vi "UHR-Fleezers Control (host) - 11.0.vi"() -> ()   [LabVIEW 2011] (continued)
        n1876 = property on="Trap Pos FB SP 2" class="DigNum (strict)"("Val(Sgnl)"=w2723) -> ()  [unwired: 2 in, 2 out]
        n1877 = local write "Offset SP2 from SP1"(FALSE ("Offset SP2 from SP1")) -> ()
      }
      event "Set Reading to\nSetpoint": Value Change {
        # "This is the actual PID input signal"
        n1878 = event-data() -> ()  [unwired: 7 out]
        n1879 = local write "Set Reading to\nSetpoint"(FALSE ("Set SP to Reading")) -> ()
        n1880 = xnode "Read/Write Control"("FPGA VI Reference In"=w2731, "error in"=w2730) -> ("FPGA VI Reference Out"=w2729:T19, "error out"=w2728:errorcluster, "Trap Pos FB Int-Norm Signal"=w2727:fxp<+/-,16,1>)
        n1881 = local read "Differential FB?"() -> (w2732:bool)
        n1882 = case shown="False" w2732 {
          tunnel: [w2737 w2744] -> w2734
          tunnel: w2727 -> [w2735 w2744]
          frame False {
            n1883 = local read "Trap Pos FB Monitor\nT1 or T2"() -> (w2740:bool)
            n1884 = local read "Trap X AI1 (DMA)"() -> (w2743:T13)
            n1885 = Unbundle By Name(w2743) -> ("Set 1"=w2742:fxp<+/-,16,1>, "Set 2"=w2741:fxp<+/-,16,1>)
            n1886 = Select(t=w2742, s=w2740, f=w2741) -> (s? t:f=w2739:fxp<+/-,16,1>)
            n1887 = Not(x="Set SP Using...") -> (.not. x?=w2736:bool)
            n1888 = Select(t=w2735, s=w2736, f=w2739) -> (s? t:f=w2737:fxp<+/-,16,1>)
          }
          frame True {
          }
        }
        n1889 = xnode "Read/Write Control"("FPGA VI Reference In"=w2729, "error in"=w2728, "Trap Pos. FB SP"=w2734) -> ()  [unwired: 2 out]
        n1890 = local write "Trap Pos FB SP"(w2734) -> ()
      }
      event "Trap Pos. FB Out Scale 2^n": Value Change {
        n1891 = event-data() -> ()  [unwired: 7 out]
        n1892 = Scale By Power Of 2(n="Trap Pos. FB Out Scale 2^n", x=ext 1.0) -> (x*2^n=w2745:ext)
        n1893 = property on="Trap Pos. FB Mult Factor" class="DigNum (strict)"("Val(Sgnl)"=w2745) -> ()  [unwired: 2 in, 2 out]
      }
      event "Trap Pos FB Int Count": Value Change {
        n1894 = event-data() -> ()  [unwired: 7 out]
        n1895 = xnode "Read/Write Control"("FPGA VI Reference In"=w2750, "error in"=w2749, "Trap Pos FB Int Count"="Trap Pos FB Int Count") -> ()  [unwired: 2 out]
      }
    }
    "error out 2" <- w1655
    n1896 = node-c288() -> ()  [unwired: 2 out]
  }
  n1897 = timed-loop "Mouse control: trap position (AOM deflection), set confocal spot from image" {
    tunnel: [w2752] -> w182
    tunnel: w1 -> [w2751]
    timing: w94 -> [_]
    timing-out: [_] -> w93
    stop <- w2752 stop-if-true
    n1898 = node-c288() -> ()  [unwired: 2 out]
    n1899 = event shown="[0] \"Pane\": Mouse Down" {
      selector: _ -> [_ _]
      dyn-events: _ -> [_ _]
      timeout: _ -> [_ _]
      tunnel: w2751 -> [w2755 _]
      event Mouse Down {
        n1900 = event-data() -> ("Time"=w2757:u32, "Coords"=w2756:T7, "Button"=w2758:u16)  [unwired: 6 out]
        n1901 = case shown="1" w2758 {
          tunnel: w2757 -> [_ _ w2864]
          tunnel: w2756 -> [_ w2795 w2862]
          tunnel: w2755 -> [_ _ w2860]
          frame 0, Default {
          }
          frame 1 {
            n1902 = property on="APD 2" class="ImageControl"() -> ("Displayed Image Position"=w2765:cluster{"Left":i32, "Top":i32})  [unwired: 2 in, 2 out]
            n1903 = property on="APD 1" class="ImageControl"() -> ("Displayed Image Position"=w2794:cluster{"Left":i32, "Top":i32})  [unwired: 2 in, 2 out]
            n1904 = property on="Detection Laser X" class="ImageControl"() -> ("Displayed Image Position"=w2791:cluster{"Left":i32, "Top":i32})  [unwired: 2 in, 2 out]
            n1905 = property on="Detection Laser Y" class="ImageControl"() -> ("Displayed Image Position"=w2790:cluster{"Left":i32, "Top":i32})  [unwired: 2 in, 2 out]
            n1906 = property on="APD 2" class="ImageControl"() -> ("Displayed Image Size"=w2764:cluster{"Width":u32, "Height":u32})  [unwired: 2 in, 2 out]
            n1907 = property on="APD 1" class="ImageControl"() -> ("Displayed Image Size"=w2792:cluster{"Width":u32, "Height":u32})  [unwired: 2 in, 2 out]
            n1908 = property on="Detection Laser X" class="ImageControl"() -> ("Displayed Image Size"=w2793:cluster{"Width":u32, "Height":u32})  [unwired: 2 in, 2 out]
            n1909 = property on="Detection Laser Y" class="ImageControl"() -> ("Displayed Image Size"=w2789:cluster{"Width":u32, "Height":u32})  [unwired: 2 in, 2 out]
            n1910 = Unbundle By Name(w2764) -> ("Width"=w2761:u32, "Height"=w2760:u32)
            n1911 = Unbundle By Name(w2765) -> ("Left"=w2763:i32, "Top"=w2762:i32)
            n1912 = Unbundle By Name(w2792) -> ("Width"=w2786:u32, "Height"=w2785:u32)
            n1913 = Unbundle By Name(w2793) -> ("Width"=w2782:u32, "Height"=w2781:u32)
            n1914 = Unbundle By Name(w2789) -> ("Width"=w2778:u32, "Height"=w2777:u32)
            n1915 = Unbundle By Name(w2794) -> ("Left"=w2788:i32, "Top"=w2787:i32)
            n1916 = Unbundle By Name(w2791) -> ("Left"=w2784:i32, "Top"=w2783:i32)
            n1917 = Unbundle By Name(w2790) -> ("Left"=w2780:i32, "Top"=w2779:i32)
            n1918 = Bundle("Left"=w2763, "Top"=w2762, "Width"=w2761, "Height"=w2760) -> (w2759:T29)  [unwired: 1 in]
            n1919 = Bundle("Left"=w2788, "Top"=w2787, "Width"=w2786, "Height"=w2785) -> (w2776:T29)  [unwired: 1 in]
            n1920 = Bundle("Left"=w2784, "Top"=w2783, "Width"=w2782, "Height"=w2781) -> (w2775:T29)  [unwired: 1 in]
            n1921 = Bundle("Left"=w2780, "Top"=w2779, "Width"=w2778, "Height"=w2777) -> (w2774:T29)  [unwired: 1 in]
            n1922 = Build Cluster Array(w2759, w2776, w2775, w2774) -> (w2773:T30)
            n1923 = for {
              tunnel: w2795 -> [w2806]
              tunnel: w2773 -> [w2807] mode=indexing
              shift-right: [w2804] -> w2771
              shift-left: TRUE -> [w2805]
              shift-right: [w2803] -> w2769
              shift-left: _ -> [w2799]
              shift-right: [w2802] -> w2768
              shift-left: _ -> [w2798]
              shift-right: [w2801] -> w2767
              shift-left: _ -> [w2797]
              shift-right: [w2800] -> w2766
              shift-left: _ -> [w2796]
              n1924 = case shown="True" w2805 {
                selector: w2805 -> [w2812 _]
                tunnel: w2807 -> [_ w2821]
                tunnel: w2806 -> [_ w2819]
                tunnel: [w2812 w2817] -> w2804
                tunnel: [w2811 w2816] -> w2803
                tunnel: [w2810 w2815] -> w2802
                tunnel: [w2809 w2814] -> w2801
                tunnel: [w2808 w2813] -> w2800
                tunnel: w2799 -> [w2811 _]
                tunnel: w2798 -> [w2810 _]
                tunnel: w2797 -> [w2809 _]
                tunnel: w2796 -> [w2808 _]
                frame False {
                }
                frame True {
                  n1925 = Unbundle(w2821) -> (w2820:T29)
                  n1926 = call "isclickinwindow.vi"("Image Param"=w2820, "Point32"=w2819) -> ("4 Y"=w2813:i32, "3 Height"=w2814:i32, "2 X"=w2815:i32, "1 Width"=w2816:i32, "In image?"=w2818:bool)  [unwired: 1 in]
                  n1927 = Not(x=w2818) -> (.not. x?=w2817:bool)
                }
              }
            }
            n1928 = Not(x=w2771) -> (.not. x?=w2770:bool)
            n1929 = case shown="True" w2770 {
              tunnel: w2768 -> [_ w2835]
              tunnel: w2766 -> [_ w2834]
              tunnel: w2769 -> [_ w2833]
              tunnel: w2767 -> [_ w2832]
              frame False {
              }
              frame True {
                w2822 = FALSE ("Get Point")
                n1930 = local read "Scan lines (y)"() -> (w2837:u64)
                n1931 = disable-structure shown="Disabled" {
                  frame Disabled {
                  }
                  frame Enabled {
                  }
                }
                n1932 = local read "Actual MCL Inc (V)"() -> (w2831:dbl)
                n1933 = local read "Scan steps (MCL)"() -> (w2836:u64)
                n1934 = Divide "Y Pix/step"(x=w2832, y=w2837) -> (x/y=w2844:dbl)
                n1935 = Divide "Y V/pix"(x=w2831, y=w2844) -> (x/y=w2843:dbl)
                n1936 = Divide "Y half step offset"(x=w2831, y=2.0) -> (x/y=w2845:dbl)
                n1937 = Divide "X pix/step"(x=w2833, y=w2836) -> (x/y=w2842:dbl)
                n1938 = Negate(x=w2845) -> (-x=w2846:dbl)
                n1939 = local read "Initial Y"() -> (w2852:dbl)
                n1940 = Multiply(x=w2834, y=w2843) -> (x*y=w2853:dbl)
                n1941 = Divide "X half step offset"(x=w2831, y=2.0) -> (x/y=w2839:dbl)
                n1942 = Divide "X V/pix"(x=w2831, y=w2842) -> (x/y=w2841:dbl)
                n1943 = Multiply(x=w2831, y=w2836) -> (x*y=w2848:dbl)
                n1944 = Compound Arithmetic op=ADD(w2846, w2853, w2852) -> (w2823:dbl)
                "Pointer Y (V)" <- w2823
                n1945 = Multiply(x=w2841, y=w2835) -> (x*y=w2850:dbl)
                n1946 = Negate(x=w2839) -> (-x=w2838:dbl)
                n1947 = local read "Initial X"() -> (w2851:dbl)
                n1948 = Negate(x=w2850) -> (-x=w2849:dbl)
                n1949 = Compound Arithmetic op=ADD(w2838, w2848, w2851, w2849) -> (w2824:dbl)
                "Pointer X (V)" <- w2824
                n1950 = case shown="True" "Set High F Confocal Spot (X-Y)" {
                  tunnel: w2824 -> [_ w2854]
                  tunnel: w2823 -> [_ w2855]
                  frame False {
                  }
                  frame True {
                    "Confocal Y 2 (V)" <- w2855
                    "Confocal X 2 (V)" <- w2854
                  }
                }
                n1951 = Or(x="Set X Only", y="Set Confocal Spot (X-Y)") -> (x .or. y?=w2827:bool)
                n1952 = Or(x="Set Confocal Spot (X-Y)", y="Set Y Only") -> (x .or. y?=w2826:bool)
                n1953 = case shown="True" w2827 {
                  tunnel: w2824 -> [_ w2856]
                  frame False {
                  }
                  frame True {
                    n1954 = property on="AO2" class="Slide (strict)"("Val(Sgnl)"=w2856) -> ()  [unwired: 2 in, 2 out]
                    "Confocal X 1 (V)" <- w2856
                  }
                }
                n1955 = case shown="True" w2826 {
                  tunnel: w2823 -> [_ w2857]
                  frame False {
                  }
                  frame True {
                    n1956 = property on="AO1" class="Slide (strict)"("Val(Sgnl)"=w2857) -> ()  [unwired: 2 in, 2 out]
                    "Confocal Y 1 (V)" <- w2857
                  }
                }
                n1957 = local write "Set High F Confocal Spot (X-Y)"(w2822) -> ()
                n1958 = local write "Set Confocal Spot (X-Y)"(w2822) -> ()
                n1959 = local write "Set X Only"(w2822) -> ()
                n1960 = local write "Set Y Only"(w2822) -> ()
              }
            }
          }
          frame 3 {
            n1961 = local read "BD 2 Frequency 1 (MHz)"() -> (w2858:dbl)
            n1962 = local read "BD 1 Frequency 1 (MHz)"() -> (w2859:dbl)
            n1963 = local write "Manipulating Trap"(TRUE ("Manipulating Trap")) -> ()
            n1964 = local write "Coords"(T7 {"Horizontal"=0, "Vertical"=0} ("Coords")) -> ()
            n1965 = while {
              tunnel: w2864 -> [w2869]
              tunnel: w2862 -> [w2868]
              tunnel: w2860 -> [w2867]
              tunnel: w2859 -> [w2866]
              tunnel: w2858 -> [w2865]
              stop <- w2870 stop-if-true
              n1966 = event shown="[0] \"Pane\": Mouse Move" {
                selector: _ -> [_ _]
                dyn-events: _ -> [_ _]
                timeout: _ -> [_ _]
                tunnel: ["Force Manip Abort" w2934] -> w2870
                tunnel: w2869 -> [w2877 _]
                tunnel: w2868 -> [w2875 _]
                tunnel: w2867 -> [w2874 _]
                tunnel: w2866 -> [w2873 _]
                tunnel: w2865 -> [w2872 _]
                event Mouse Move {
                  n1967 = event-data() -> ("Time"=w2878:u32, "Coords"=w2879:T7)  [unwired: 3 out]
                  n1968 = Less?(x=w2878, y=w2877) -> (x < y?=w2876:bool)
                  n1969 = case "Makes sure old motion events prior to mouse click aren't used" shown="False" w2876 {
                    tunnel: w2879 -> [w2921 _]
                    tunnel: w2875 -> [w2922 _]
                    tunnel: w2874 -> [w2899 _]
                    tunnel: w2873 -> [w2895 _]
                    tunnel: w2872 -> [w2894 _]
                    frame False {
                      n1970 = Subtract(x=w2921, y=w2922) -> (x-y=w2920:T7)
                      "Coords" <- w2920
                      n1971 = local read "Y RF Frequency Limits (MHz)"() -> (w2880:T16)
                      n1972 = To Double Precision Float(number=w2920) -> (double precision float=w2919:cluster{"Horizontal":dbl, "Vertical":dbl})
                      n1973 = Multiply(x=cluster{"Horizontal":dbl, "Vertical":dbl} {"Horizontal"=-1.0, "Vertical"=1.0}, y="Manipulation Scaling") -> (x*y=w2915:cluster{"Horizontal":dbl, "Vertical":dbl})
                      n1974 = local read "X RF Frequency Limits (MHz)"() -> (w2881:T16)
                      n1975 = Multiply(x=w2919, y=w2915) -> (x*y=w2917:cluster{"Horizontal":dbl, "Vertical":dbl})
                      n1976 = Unbundle By Name(w2917) -> ("Horizontal"=w2912:dbl, "Vertical"=w2916:dbl)
                      n1977 = Unbundle By Name(w2880) -> ("Maximum"=w2883:dbl, "Minimum"=w2882:dbl)
                      n1978 = Boolean To (0,1)(Boolean="Manip. X?") -> (0, 1=w2910:i16)
                      n1979 = Boolean To (0,1)(Boolean="Manip. Y?") -> (0, 1=w2907:i16)
                      n1980 = local read "BD 1 Frequency 2 (MHz)"() -> (w2897:dbl)
                      n1981 = Multiply(x=w2916, y=w2907) -> (x*y=w2909:dbl)
                      n1982 = Multiply(x=w2910, y=w2912) -> (x*y=w2913:dbl)
                      n1983 = local read "BD 2 Frequency 2 (MHz)"() -> (w2896:dbl)
                      n1984 = Unbundle By Name(w2881) -> ("Maximum"=w2885:dbl, "Minimum"=w2884:dbl)
                      n1985 = Add(x=w2894, y=w2909) -> (x+y=w2887:dbl)
                      n1986 = Add(x=w2895, y=w2913) -> (x+y=w2889:dbl)
                      n1987 = In Range and Coerce(upper limit=w2885, x=w2889, lower limit=w2884) -> (coerced(x)=w2888:dbl)  [unwired: 1 out]
                      n1988 = In Range and Coerce(upper limit=w2883, x=w2887, lower limit=w2882) -> (coerced(x)=w2886:dbl)  [unwired: 1 out]
                      n1989 = Subtract(x=w2888, y=w2897) -> (x-y=w2906:dbl)
                      n1990 = Subtract(x=w2886, y=w2896) -> (x-y=w2905:dbl)
                      n1991 = Square(x=w2906) -> (x^2=w2904:dbl)
                      n1992 = Square(x=w2905) -> (x^2=w2903:dbl)
                      n1993 = Add(x=w2904, y=w2903) -> (x+y=w2902:dbl)
                      n1994 = Square Root(x=w2902) -> (sqrt(x)=w2898:dbl)
                      n1995 = In Range and Coerce(upper limit="Limit Max (MHz)", x=w2898, lower limit="Limit Min (MHz)") -> (In Range?=w2891:bool)  [unwired: 1 out]
                      n1996 = Not(x="Limits Enable") -> (.not. x?=w2890:bool)
                      n1997 = Or(x=w2891, y=w2890) -> (x .or. y?=w2892:bool)
                      n1998 = case shown="True" w2892 {
                        tunnel: w2899 -> [_ w2932]
                        tunnel: w2898 -> [_ w2923]
                        tunnel: w2888 -> [_ w2930]
                        tunnel: w2897 -> [_ w2929]
                        tunnel: w2886 -> [_ w2928]
                        tunnel: w2896 -> [_ w2927]
                        tunnel: w2881 -> [_ w2925]
                        tunnel: w2880 -> [_ w2924]
                        frame False {
                        }
                        frame True {
                          n1999 = local read "BD 1 Frequency 3 (MHz)"() -> (w2931:dbl)
                          n2000 = local read "BD 2 Frequency 3 (MHz)"() -> (w2926:dbl)
                          n2001 = local write "Trap Delta (MHz)"(w2923) -> ()
                          n2002 = call "set RF board frequency - interlace.vi"("Board 2 Frequency Limits"=w2924, "Board 1 Frequency Limits"=w2925, "FPGA VI Reference In"=w2932, "Board 2 Frequency 3 (MHz)"=w2926, "Board 1 Frequency 3 (MHz)"=w2931, "Board 2 Frequency 2 (MHz)"=w2927, "Board 2 Frequency 1 (MHz)"=w2928, "Board 1 Frequency 2 (MHz)"=w2929, "Board 1 Frequency 1  (MHz)"=w2930) -> ()  [unwired: 1 in, 2 out]
                          n2003 = local write "BD 2 Frequency 1 (MHz)"(w2928) -> ()
                          n2004 = local write "BD 1 Frequency 1 (MHz)"(w2930) -> ()
                        }
                      }
                    }
                    frame True {
                    }
                  }
                }
                event Mouse Up {
                  n2005 = event-data() -> ("Button"=w2933:u16)  [unwired: 8 out]
                  n2006 = case shown="3" w2933 {
                    tunnel: [FALSE TRUE] -> w2934
                    frame 0, Default {
                    }
                    frame 3 {
                      n2007 = local read "Trap Delta (MHz)"() -> (w2936:dbl)
                      n2008 = property on="Initial delta (MHz)" class="DigNum (strict)"("Val(Sgnl)"=w2936) -> ()  [unwired: 2 in, 2 out]
                      n2009 = local write "Manipulating Trap"(FALSE ("Manipulating Trap")) -> ()
                    }
                  }
                }
              }
            }
          }
        }
      }
      event Mouse Move {
        n2010 = event-data() -> ()  [unwired: 6 out]
      }
    }
    n2011 = local read "Stop All"() -> (w2752:bool)
    n2012 = node-c288() -> ()  [unwired: 2 out]
  }
  n2013 = node-c288(w91) -> ()  [unwired: 1 out]
  n2014 = node-c288(w93) -> ()  [unwired: 1 out]
  n2015 = node-c288(w78) -> ()  [unwired: 1 out]
  n2016 = flat-sequence "Video" {
    tunnel: [w2947] -> w80
    tunnel: w80 -> [w2988]
    frame #0 {
      n2017 = while {
        stop <- w2940 continue-if-true
        n2018 = call "Close Video Capture.vi"() -> ("error code OUT"=w2942:i32)
        n2019 = Equal?(x=w2942, y=0) -> (x = y?=w2940:bool)
      }
      n2020 = local write "Stop All"(FALSE ("Stop All")) -> ()
    }
    frame #1 {
      n2021 = call "DMR_Init.vi"() -> ()  [unwired: 3 out]
    }
    frame #2 {
      # "Setting the destination format to Mono8 makes sure that the image can be displayed in the intensity plot."
      n2022 = call "DMR_GetDevice.vi"("search string IN"="DE019116701") -> ("device handle OUT"=w2965:i32)  [unwired: 4 in, 2 out]
      n2023 = call "DMR_OpenDevice.vi"("device handle IN"=w2965) -> ("driver handle OUT"=w2948:i32)  [unwired: 4 out]
      n2024 = call "DMR_FindList.vi"("flags IN"=u32 0 ("flags"), "list name IN"="" ("String"), "list type IN"=T31."camera descriptions", "driver handle IN"=w2948) -> ("list handle OUT"=w2951:i32)  [unwired: 2 out]
      n2025 = call "DMR_FindList.vi"("flags IN"=u32 0 ("flags"), "list name IN"="Base", "list type IN"=T31."setting", "driver handle IN"=w2948) -> ("list handle OUT"=w2949:i32)  [unwired: 2 out]
      n2026 = call "OBJ_GetHandle.vi"("object name IN"="VideoStandard", "list handle IN"=w2951) -> ("object handle OUT"=w2945:i32)  [unwired: 3 out]
      n2027 = call "OBJ_GetHandle.vi"("object name IN"="PixelFormat", "list handle IN"=w2949) -> ("object handle OUT"=w2959:i32)  [unwired: 3 out]
      n2028 = call "OBJ_SetS.vi"("value index IN"=0, "value IN"="NTSC M", "object handle IN"=w2945) -> ()  [unwired: 2 out]
      n2029 = call "OBJ_SetS.vi"("value index IN"=0, "value IN"="Mono8" ("value"), "object handle IN"=w2959) -> ()  [unwired: 2 out]
      n2030 = call "OBJ_GetHandle.vi"("object name IN"="VideoChannel", "list handle IN"=w2949) -> ("object handle OUT"=w2955:i32)  [unwired: 3 out]
      n2031 = while {
        tunnel: [w2970] -> w2947
        tunnel: w2948 -> [w2967]
        stop <- w2968 continue-if-true
        n2032 = call "DMR_ImageRequestSingle.vi"("request control IN"=0, "driver handle IN"=w2967) -> ("error code OUT"=w2969:i32, "driver handle OUT"=w2970:i32)  [unwired: 2 out]
        n2033 = Equal To 0?(x=w2969) -> (x = 0?=w2968:bool)
      }
      n2034 = call "OBJ_SetI.vi"("value index IN"=0, "value IN"=3 ("Video channel"), "object handle IN"=w2955) -> ()  [unwired: 2 out]
    }
    frame #3 {
      w2976 = T17 0 items=["Grayscale (U8)", "Grayscale (I16)", "Grayscale (SGL)", "Complex (CSG)", "RGB (U32)", "HSL (U32)", "RGB (U64)"] ("Image Type")
      w2984 = T17 0 items=["Grayscale (U8)", "Grayscale (I16)", "Grayscale (SGL)", "Complex (CSG)", "RGB (U32)", "HSL (U32)", "RGB (U64)"] ("Image Type")
      n2035 = for "Create Greyscale map" {
        N: 256 -> [_]
        tunnel: [w2990] -> w2973 mode=indexing
        workers-P: _ -> [_]
        i -> [w2993]
        n2036 = To Unsigned Byte Integer(number=w2993) -> (unsigned 8bit integer=w2989:u8)
        n2037 = Join Numbers(hi=w2989, lo=w2989) -> ((hi.lo)=w2992:u16)
        n2038 = Join Numbers(hi=w2989, lo=w2989) -> ((hi.lo)=w2991:u16)
        n2039 = Join Numbers(hi=w2992, lo=w2991) -> ((hi.lo)=w2990:u32)
      }
      n2040 = call "IMAQ Create"("Image Name"="Scaled video", "Image Type"=w2976) -> ("New Image"=w2975:T2)  [unwired: 2 in, 2 out]
      n2041 = call "IMAQ Create"("Image Name"="Main video", "Image Type"=w2984) -> ("New Image"=w2985:T2)  [unwired: 2 in, 2 out]
      n2042 = node-c288(0 ("Processor")) -> (w2983:T21)  [unwired: 3 out]
      n2043 = Initialize Array(u32 0 ("Window Number (0...15)"), 480 ("dimension size"), 640 ("dimension size")) -> (w2978:u32[][])
      n2044 = timed-loop {
        tunnel: w2988 -> [w3010]
        tunnel: [w3009] -> w2987
        tunnel: w2985 -> [w3008]
        timing: w2983 -> [_]
        timing-out: [_] -> w2982
        tunnel: w2978 -> [w2997]
        tunnel: w2975 -> [w2995]
        tunnel: w2973 -> [w2994]
        stop <- w2996 stop-if-true
        # "This block performs the \nactual image capture."
        n2045 = node-c288() -> ()  [unwired: 2 out]
        n2046 = local read "Stop All"() -> (w2996:bool)
        n2047 = Reciprocal(x="Video Capture Rate (Hz)") -> (1/x=w3000:dbl)
        n2048 = Multiply(x=w3000, y=1000.0) -> (x*y=w2998:dbl)
        n2049 = call "DMR_ImageRequestWaitFor.vi"("queue number IN"=0, "timeout(ms) IN"=500, "driver handle IN"=w3010) -> ("error code OUT"=w3014:i32, "request number OUT"=w3011:i32, "driver handle OUT"=w3012:i32)
        n2050 = feedback #1(T32 refnum ("Avi Refnum")) -> (w3002:T32)
        n2051 = case shown="True" "New Video File" {
          tunnel: [T32 refnum ("Avi Refnum") w3031] -> w3004
          tunnel: [FALSE TRUE] -> w3005
          tunnel: w3002 -> [_ w3027]
          frame False {
          }
          frame True {
            n2052 = call "Create new save file.vi"("Ext"=".avi" ("string"), "Index In"="Video Index") -> ("Path Out"=w3023:path, "Index Out"=w3024:dbl)  [unwired: 1 in]
            "Path Out" <- w3023
            n2053 = Not Equal?(x=w3027, y=T32 refnum ("Avi Refnum")) -> (x != y?=w3028:bool)
            n2054 = Increment(x=w3024) -> (x+1=w3033:dbl)
            n2055 = case shown="True" w3028 {
              tunnel: w3027 -> [_ w3034]
              frame False {
              }
              frame True {
                n2056 = call "IMAQ AVI Close"("Avi Refnum"=w3034) -> ()  [unwired: 1 in, 10 out]
              }
            }
            n2057 = local write "Video Index"(w3033) -> ()
            n2058 = call "IMAQ AVI Create"("Frames Per Second"=u32 30, "AVI Path"=w3023) -> ("Avi Refnum"=w3031:T32)  [unwired: 5 in, 4 out]
          }
        }
        n2059 = Equal To 0?(x=w3014) -> (x = 0?=w3013:bool)
        n2060 = Select(t=w3004, s=w3005, f=w3002) -> (s? t:f=w3003:T32)
        n2061 = feedback-in #1(w3003) -> ()
        n2062 = case shown="True" w3013 {
          tunnel: w3012 -> [w3035 w3060]
          tunnel: w3011 -> [_ w3059]
          tunnel: [w3035 w3056] -> w3009
          tunnel: w3008 -> [_ w3040]
          tunnel: w2997 -> [_ w3044]
          tunnel: w3003 -> [_ w3042]
          tunnel: w2995 -> [_ w3037]
          tunnel: w2994 -> [_ w3036]
          frame False {
          }
          frame True {
            w3050 = u32 0 ("X-offset IN")
            n2063 = call "DMR_GetImageRequestBufferData.vi"("driver handle IN"=w3060, "request number IN"=w3059) -> ("width OUT"=w3049:i32, "height OUT"=w3048:i32, "driver handle OUT"=w3055:i32, "request number OUT"=w3054:i32, "bytes per pixel OUT"=w3051:i32)  [unwired: 13 out]
            n2064 = call "DMR_GetImageRequestBufferImageData.vi"("driver handle IN"=w3055, "request number IN"=w3054, "bytes per pixel IN"=w3051, "X-offset IN"=w3050, "Y-offset IN"=w3050, "height IN"=w3048, "width IN"=w3049) -> ("driver handle OUT"=w3053:u32, "request number OUT"=w3052:u32, "image OUT"=w3045:u32[][])  [unwired: 10 out]
            n2065 = call "DMR_ImageRequestUnlock.vi"("request number IN"=w3052, "driver handle IN"=w3053) -> ("driver handle OUT"=w3058:i32)  [unwired: 1 in, 2 out]
            n2066 = case shown="True" "Averaging" {
              tunnel: w3045 -> [w3096 w3101]
              tunnel: [w3096 w3100] -> w3041
              tunnel: w3044 -> [_ w3098]
              frame False {
              }
              frame True {
                (unwired) 1
                w3106 = 1
                n2067 = feedback #2(w3098) -> (w3097:u32[][])
                n2068 = Add(x=w3101, y=w3097) -> (x+y=w3102:u32[][])
                n2069 = Select(t=w3098, s="Reset Averaging", f=w3102) -> (s? t:f=w3104:u32[][])
                n2070 = feedback-in #2(w3104) -> ()
                n2071 = feedback #3(w3106) -> (w3099:i32)
                n2072 = Divide(x=w3102, y=w3099) -> (x/y=w3103:dbl[][])
                n2073 = Increment(x=w3099) -> (x+1=w3107:i32)
                n2074 = To Unsigned Long Integer(number=w3103) -> (unsigned 32bit integer=w3100:u32[][])
                n2075 = Select(t=w3106, s="Reset Averaging", f=w3107) -> (s? t:f=w3105:i32)
                n2076 = feedback-in #3(w3105) -> ()
              }
            }
            n2077 = call "DMR_ImageRequestSingle.vi"("request control IN"=0, "driver handle IN"=w3058) -> ("driver handle OUT"=w3056:i32)  [unwired: 3 out]
            n2078 = disable-structure shown="Disabled" {
              disable-tunnel: w3041 -> [w3073 _]
              disable-tunnel: w3037 -> [w3072 _]
              frame Disabled {
                n2079 = To Double Precision Float(number=w3073) -> (double precision float=w3071:dbl[][])
                n2080 = In Range and Coerce(upper limit="Intensity Upper", x=w3071, lower limit="Intensity Lower") -> (coerced(x)=w3070:dbl[][])  [unwired: 1 out]
                n2081 = Subtract(x="Intensity Upper", y="Intensity Lower") -> (x-y=w3067:dbl)
                n2082 = Subtract(x=w3070, y="Intensity Lower") -> (x-y=w3068:dbl[][])
                n2083 = Divide(x=w3068, y=w3067) -> (x/y=w3069:dbl[][])
                n2084 = Multiply(x=255.0, y=w3069) -> (x*y=w3065:dbl[][])
                n2085 = To Unsigned Byte Integer(number=w3065) -> (unsigned 8bit integer=w3074:u8[][])
                n2086 = call "IMAQ ArrayToImage"("Image Pixels (U8)"=w3074, "Image"=w3072) -> ("Image Out"=w3061:T2)  [unwired: 4 in, 5 out]
                n2087 = First Call?() -> (First Call?: T/F=w3062:bool)
                n2088 = case shown="True" w3062 {
                  tunnel: w3061 -> [w3075 w3086]
                  frame False {
                    n2089 = flat-sequence {
                      tunnel: w3075 -> [w3081]
                      frame #0 {
                        w3078 = FALSE ("Get/Set Status? (Set)")
                        w3077 = 0 ("Window Number (0...15)")
                        n2090 = call "IMAQ WindSize"("Get/Set Status? (Set)"=w3078, "Window Number"=w3077) -> ("Width & Height out"=→"Window Size":cluster{"Width":i32, "Height":i32})  [unwired: 4 in, 2 out]
                        n2091 = call "IMAQ WindMove"("Window Number (0...15)"=w3077, "Get/Set Status? (Set)"=w3078) -> ("Coordinates (screen)"=→"Window Position":cluster{"X Position":i32, "Y Position":i32})  [unwired: 3 in, 1 out]
                        n2092 = call "IMAQ WindDraw"("Resize to Image Size? (Y)"=FALSE, "Window Number (0...15)"=w3077, "Image"=w3081) -> ()  [unwired: 7 in, 2 out]
                      }
                      frame #1 {
                        n2093 = call "IMAQ WindZoom 2"("Center Point"="Center Point", "Zoom to Fit? (False)"=FALSE, "Zoom Factor"="Zoom Factor") -> ()  [unwired: 5 in, 4 out]
                      }
                    }
                  }
                  frame True {
                    n2094 = flat-sequence {
                      tunnel: w3086 -> [w3089]
                      tunnel: [w3087] -> w3085
                      tunnel: w3085 -> [w3091]
                      frame #0 {
                        w3088 = TRUE ("Resize to Image Size? (Y)")
                        w3087 = 0 ("Window Number (0...15)")
                        n2095 = call "IMAQ WindNonTearing"("Window Number"=w3087, "NonTearing? (True)"=w3088) -> ()  [unwired: 8 in, 2 out]
                        n2096 = call "IMAQ WindDraw"("Resize to Image Size? (Y)"=w3088, "Window Number (0...15)"=w3087, "Image"=w3089) -> ()  [unwired: 7 in, 2 out]
                      }
                      frame #1 {
                        n2097 = call "IMAQ WindSize"("Scrollbars? (N)"=FALSE, "Width & Height"="Initial Window Size", "Window Number"=w3091) -> ()  [unwired: 3 in, 3 out]
                        n2098 = call "IMAQ WindMove"("Window Number (0...15)"=w3091, "Coordinates (screen)"="Initial Window Position") -> ()  [unwired: 3 in, 2 out]
                      }
                    }
                  }
                }
              }
              frame Enabled {
              }
            }
            n2099 = To Unsigned Byte Integer(number=w3041) -> (unsigned 8bit integer=w3039:u8[][])
            n2100 = call "IMAQ ArrayToImage"("Image Pixels (U8)"=w3039, "Image"=w3040) -> ("Image Out"=w3038:T2)  [unwired: 4 in, 5 out]
            "Primary Video Display" <- w3038
            n2101 = case shown="True" "Save Video" {
              tunnel: w3042 -> [_ w3095]
              tunnel: w3038 -> [_ w3094]
              frame False {
              }
              frame True {
                n2102 = call "IMAQ AVI Write Frame"("Image"=w3094, "Avi Refnum"=w3095) -> ()  [unwired: 2 in, 8 out]
              }
            }
            n2103 = case shown="True" "Save Image" {
              tunnel: w3039 -> [_ w3110]
              tunnel: w3036 -> [_ w3109]
              frame False {
              }
              frame True {
                n2104 = call <vilib>:"Flatten Pixmap.vi"("colors"=w3109, "8-bit pixmap"=w3110) -> ("image data"=w3116:T33)  [unwired: 4 in, 5 out]
                n2105 = call "Create new save file.vi"("Insert"="video_frame_" ("string"), "Ext"=".bmp" ("string"), "Index In"="Image Index") -> ("Path Out"=w3112:path, "Index Out"=w3117:dbl)
                n2106 = Increment(x=w3117) -> (x+1=w3111:dbl)
                n2107 = local write "Image Index"(w3111) -> ()
                n2108 = call <vilib>:"Write BMP File.vi"("image data"=w3116, "path to BMP file"=w3112) -> ()  [unwired: 1 in, 9 out]
              }
            }
          }
        }
        n2109 = node-c288(w2998) -> ()  [unwired: 1 out]
      }
      n2110 = node-c288(w2982) -> ()  [unwired: 1 out]
      n2111 = call "DMR_CloseDevice.vi"("driver handle IN"=w2987) -> ()  [unwired: 1 in, 4 out]
    }
    frame #4 {
      n2112 = call "DMR_Close.vi"() -> ()  [unwired: 1 out]
    }
  }
  n2113 = node-c288(i64 1 ("Period"), 1 ("Processor")) -> (w175:T21)  [unwired: 2 out]
  n2114 = timed-loop "Acquire Data" {
    tunnel: w1 -> [w3416]
    tunnel: w50 -> [w3415]
    tunnel: [w3445] -> w270
    tunnel: [w3440] -> w268
    timing: w175 -> [_]
    timing-out: [_] -> w174
    tunnel: w69 -> [w3253]
    stop <- "Stop All" stop-if-true
    w3168 = "Initialize"
    w3238 = "NI_ChannelName" ("name")
    n2115 = node-c288() -> ()  [unwired: 2 out]
    n2116 = First Call?() -> (First Call?: T/F=w3203:bool)
    n2117 = Or(x="Reset", y=w3203) -> (x .or. y?=w3204:bool)
    n2118 = local read "Flushing P1"() -> (w3122:bool)
    n2119 = case "Reset data stream" shown="True" w3204 {
      tunnel: w3416 -> [w4421 w4429]
      tunnel: w3415 -> [w4420 w4428]
      tunnel: [w4421 w4423] -> w3411
      tunnel: [w4420 w4422] -> w3410
      frame False {
      }
      frame True {
        w4426 = TRUE ("AI to FIFO")
        n2120 = local write "Overflow (data lost)"(FALSE ("Overflow (data lost)")) -> ()
        n2121 = call "reset FPGA DMA.vi"("error in"=w4428, "FPGA VI Reference In"=w4429) -> ("error out"=w4424:errorcluster, "FPGA VI Reference Out"=w4425:T19)
        n2122 = xnode "Read/Write Control"("FPGA VI Reference In"=w4425, "error in"=w4424, "AI to FIFO"=w4426, "APD to FIFO"=w4426) -> ("FPGA VI Reference Out"=w4423:T19, "error out"=w4422:errorcluster)
      }
    }
    n2123 = case shown="True" w3122 {
      frame False {
      }
      frame True {
        n2124 = local read "Flush rate (uL/m) P1"() -> (w3462:dbl)
        n2125 = local read "HP1 Flush Time (s)"() -> (w3471:dbl)
        n2126 = local read "DMA Update Period (s)"() -> (w3465:dbl)
        n2127 = Divide(x=w3462, y=60.0) -> (x/y=w3463:dbl)
        n2128 = Divide(x=w3471, y=w3465) -> (x/y=w3460:dbl)
        n2129 = feedback #4(0) -> (w3469:i32)
        n2130 = Increment(x=w3469) -> (x+1=w3459:i32)
        n2131 = Greater?(x=w3459, y=w3460) -> (0:w3468:bool)
        n2132 = Compound Arithmetic op=MULTIPLY(w3465, w3459, w3463) -> (→"P1 Flush Volume (uL)":dbl)
        n2133 = Divide(x=w3459, y=w3460) -> (x/y=→"P1 Flushing Bar":dbl)
        n2134 = case shown="True" w3468 {
          tunnel: w3459 -> [w3472 _]
          tunnel: [w3472 0] -> w3467
          frame False {
          }
          frame True {
            w3473 = FALSE ("Flushing P1")
            n2135 = local write "Inject Pump 1"(w3473) -> ()
            n2136 = local write "Flushing P1"(w3473) -> ()
            n2137 = property on="Clear Volume P1" class="Bool (strict)"("Val(Sgnl)"=TRUE ("Value (Signaling)")) -> ()  [unwired: 2 in, 2 out]
          }
        }
        n2138 = feedback-in #4(w3467) -> ()
      }
    }
    n2139 = Or(x="Start AOD Scan", y="Trap Raster Scan") -> (x .or. y?=w3361:bool)
    n2140 = case "Start AOM raster scan" shown="True" w3361 {
      tunnel: w3411 -> [w4271 w4281]
      tunnel: w3410 -> [w4270 w4280]
      tunnel: [w4271 w4274] -> w3409
      tunnel: [w4270 w4273] -> w3408
      frame False {
      }
      frame True {
        n2141 = case shown="True" "Restart DMA? (AOD)" {
          tunnel: [w4319 w4321] -> w4275
          tunnel: [w4318 w4320] -> w4276
          tunnel: w4281 -> [w4319 w4323]
          tunnel: w4280 -> [w4318 w4322]
          frame False {
          }
          frame True {
            n2142 = local write "Overflow (data lost)"(FALSE ("Overflow (data lost)")) -> ()
            n2143 = call "reset FPGA DMA.vi"("error in"=w4322, "FPGA VI Reference In"=w4323) -> ("error out"=w4320:errorcluster, "FPGA VI Reference Out"=w4321:T19)
          }
        }
        n2144 = local write "Trap Raster Scan"(FALSE ("Trap Raster Scan")) -> ()
        n2145 = case shown="True" "Move MCL Also?" {
          tunnel: w4276 -> [w4284 w4313]
          tunnel: w4275 -> [w4285 w4314]
          tunnel: [w4283 w4317] -> w4274
          tunnel: [w4282 w4316] -> w4273
          frame False {
            w4286 = TRUE ("AI to FIFO")
            n2146 = xnode "Read/Write Control"("FPGA VI Reference In"=w4285, "error in"=w4284, "AI to FIFO"=w4286, "APD to FIFO"=w4286, "Start scan"=w4286) -> ("FPGA VI Reference Out"=w4283:T19, "error out"=w4282:errorcluster)
          }
          frame True {
            w4310 = FALSE ("1D or 2D Scan?")
            w4315 = TRUE ("AI to FIFO")
            # "Count for MCL loop"
            # "N total cycles"
            # "N steps"
            # "V_int"
            n2147 = local read "Scan Range (nm)"() -> (w4292:dbl)
            n2148 = local read "Number of F/B Scans (AOD)"() -> (w4309:u16)
            n2149 = Sign(1:w4292) -> (0:w4291:dbl)
            n2150 = Compound Arithmetic op=MULTIPLY(w4292, "MCL Step Position Ratio", "MCL/AOM Scale Tweak") -> (w4296:dbl)
            n2151 = Negate(x=w4291) -> (-x=w4288:dbl)
            n2152 = Multiply(x=w4288, y="MCL Step Increment (V_int)") -> (x*y=w4290:dbl)
            n2153 = Divide(x=w4296, y="MCL X Cal (nm/V)") -> (x/y=w4302:dbl)
            n2154 = Multiply(x=32767.0 ("y"), y=w4302) -> (x*y=w4308:dbl)
            n2155 = local read "Total Counts (ticks)"() -> (w4293:u32)
            n2156 = local read "Cycles/step (AOD)"() -> (w4304:u64)
            n2157 = local read "Scan steps (AOD)"() -> (w4305:u64)
            n2158 = Divide(x=w4308, y=10.0) -> (x/y=w4301:dbl)
            n2159 = Divide(x=w4301, y="MCL Step Increment (V_int)") -> (x/y=w4299:dbl)
            n2160 = Absolute Value(x=w4299) -> (abs(x)=w4287:dbl)
            n2161 = Compound Arithmetic op=MULTIPLY(w4305, w4304, w4293) -> (w4300:u64)
            n2162 = local write "wait to reset values"(w4315) -> ()
            n2163 = local write "MCL Scanning"(w4315) -> ()
            n2164 = Divide(x=w4300, y=w4287) -> (x/y=w4297:dbl)
            "MCL Count" <- w4297
            n2165 = xnode "Read/Write Control"("FPGA VI Reference In"=w4314, "error in"=w4313, "Scan steps (MCL)"=w4287, "Number of scans (MCL)"=w4309, "Cycles per step (MCL)"=u64 1, "Scan freq.  increment (MCL)"=w4290, "1D or 2D Scan?"=w4310, "MCL Scan Axis"=w4310, "Cont. Scan (MCL)"=w4310, "MCL count"=w4297) -> ("FPGA VI Reference Out"=w4312:T19, "error out"=w4311:errorcluster)
            n2166 = xnode "Read/Write Control"("FPGA VI Reference In"=w4312, "error in"=w4311, "AI to FIFO"=w4315, "APD to FIFO"=w4315, "Start scan"=w4315, "Start scan (MCL)"=w4315) -> ("FPGA VI Reference Out"=w4317:T19, "error out"=w4316:errorcluster)
          }
        }
        "Raster Scanning..." <- TRUE ("Scanning...")
      }
    }
    n2167 = local read "Flushing P3"() -> (w3123:bool)
    n2168 = case "Keep track of when Harvard Pump 3 is done flushing" shown="True" w3123 {
      frame False {
      }
      frame True {
        n2169 = local read "Flush rate (uL/m) P3"() -> (w3479:dbl)
        n2170 = local read "DMA Update Period (s)"() -> (w3481:dbl)
        n2171 = local read "HP3 Flush Time (s)"() -> (w3488:dbl)
        n2172 = Divide(x=w3479, y=60.0) -> (x/y=w3477:dbl)
        n2173 = feedback #5(0) -> (w3486:i32)
        n2174 = Increment(x=w3486) -> (x+1=w3480:i32)
        n2175 = Divide(x=w3488, y=w3481) -> (x/y=w3482:dbl)
        n2176 = Greater?(x=w3480, y=w3482) -> (0:w3485:bool)
        n2177 = Compound Arithmetic op=MULTIPLY(w3481, w3480, w3477) -> (→"P3 Flush Volume (uL)":dbl)
        n2178 = case shown="True" w3485 {
          tunnel: w3480 -> [w3489 _]
          tunnel: [w3489 0] -> w3484
          frame False {
          }
          frame True {
            w3490 = FALSE ("Flushing P3")
            n2179 = local write "Inject Pump 3"(w3490) -> ()
            n2180 = local write "Flushing P3"(w3490) -> ()
            n2181 = property on="Clear Volume P3" class="Bool (strict)"("Val(Sgnl)"=TRUE ("Value (Signaling)")) -> ()  [unwired: 2 in, 2 out]
          }
        }
        n2182 = feedback-in #5(w3484) -> ()
        n2183 = Divide(x=w3480, y=w3482) -> (x/y=→"P3 Flushing Bar":dbl)
      }
    }
    n2184 = And(x="Save scans", y=w3361) -> (x .and. y?=w3407:bool)
    n2185 = Compound Arithmetic op=OR("Start MCL Scan", "Confocal Image", "Confocal Linescan") -> (w3359:bool)
    n2186 = And(x="Save Data (MCL)", y=w3359) -> (x .and. y?=w3406:bool)
    n2187 = case "Start MCL raster scan" shown="True" w3359 {
      tunnel: w3409 -> [w3888 w3904]
      tunnel: w3408 -> [w3887 w3903]
      tunnel: [w3888 w3899] -> w3251
      tunnel: [w3887 w3898] -> w3250
      tunnel: [FALSE w3897] -> w3392
      tunnel: "Start MCL Scan" -> [_ w3892]
      tunnel: "Confocal Image" -> [_ w3891]
      tunnel: "Confocal Linescan" -> [_ _]
      frame False {
      }
      frame True {
        w3897 = TRUE
        n2188 = case shown="True" "Restart DMA? (MCL)" {
          tunnel: [w3949 w3951] -> w3902
          tunnel: [w3948 w3950] -> w3901
          tunnel: w3904 -> [w3949 w3954]
          tunnel: w3903 -> [w3948 w3953]
          frame False {
          }
          frame True {
            n2189 = call "reset FPGA DMA.vi"("error in"=w3953, "FPGA VI Reference In"=w3954) -> ("error out"=w3950:errorcluster, "FPGA VI Reference Out"=w3951:T19)
            n2190 = local write "Overflow (data lost)"(FALSE ("Overflow (data lost)")) -> ()
          }
        }
        n2191 = case shown="False" w3892 {
          selector: w3892 -> [_ w3908]
          tunnel: w3891 -> [w3907 _]
          tunnel: [w3907 w3908] -> w3890
          frame False {
            n2192 = property on="2D or 1D Scan" class="Bool (strict)"("Val(Sgnl)"=w3907) -> ()  [unwired: 2 in, 2 out]
            n2193 = property on="Confocal Image" class="Bool (strict)"("Value"=FALSE ("Start Confocal Map")) -> ()  [unwired: 2 in, 2 out]
          }
          frame True {
          }
        }
        n2194 = local write "MCL Scanning"(w3897) -> ()
        n2195 = local read "AO1"() -> (w3894:dbl)
        n2196 = local read "AO2"() -> (w3893:dbl)
        n2197 = case shown="True" "Center Scan" {
          tunnel: w3902 -> [w3915 w3947]
          tunnel: w3901 -> [w3914 w3946]
          tunnel: [w3913 w3945] -> w3899
          tunnel: [w3912 w3944] -> w3898
          tunnel: [w3910 w3931] -> w3896
          tunnel: [w3909 w3930] -> w3895
          tunnel: w3894 -> [w3910 w3936]
          tunnel: w3893 -> [w3909 w3939]
          tunnel: w3890 -> [_ _]
          frame False {
            w3911 = TRUE ("AI to FIFO")
            n2198 = xnode "Read/Write Control"("FPGA VI Reference In"=w3915, "error in"=w3914, "AI to FIFO"=w3911, "APD to FIFO"=w3911, "Start scan (MCL)"=w3911) -> ("FPGA VI Reference Out"=w3913:T19, "error out"=w3912:errorcluster)
          }
          frame True {
            w3943 = TRUE ("AI to FIFO")
            n2199 = local read "Scan steps (MCL)"() -> (w3922:u64)
            n2200 = local read "Scan lines (y)"() -> (w3918:u64)
            n2201 = local read "Fast Scan Dir"() -> (w3929:bool)
            n2202 = local read "Actual MCL Inc (V)"() -> (w3919:dbl)
            n2203 = Decrement(x=w3918) -> (x-1=w3917:u64)
            n2204 = Decrement(x=w3922) -> (x-1=w3921:u64)
            n2205 = Multiply(x=w3919, y=w3917) -> (x*y=w3916:dbl)
            n2206 = Divide(x=w3916, y=2.0) -> (x/y=w3926:dbl)
            n2207 = Multiply(x=w3919, y=w3921) -> (x*y=w3920:dbl)
            n2208 = Divide(x=w3920, y=2.0) -> (x/y=w3925:dbl)
            n2209 = Select(t=w3925, s=w3929, f=w3926) -> (s? t:f=w3924:dbl)
            n2210 = Select(t=w3926, s=w3929, f=w3925) -> (s? t:f=w3928:dbl)
            n2211 = Subtract(x=w3936, y=w3928) -> (x-y=w3927:dbl)
            n2212 = Subtract(x=w3939, y=w3924) -> (x-y=w3923:dbl)
            n2213 = local read "2D or 1D Scan"() -> (w3941:bool)
            n2214 = Not(x=w3929) -> (.not. x?=w3935:bool)
            n2215 = Not(x=w3941) -> (.not. x?=w3937:bool)
            n2216 = And(x=w3929, y=w3937) -> (x .and. y?=w3938:bool)
            n2217 = And(x=w3937, y=w3935) -> (x .and. y?=w3940:bool)
            n2218 = Select(t=w3939, s=w3940, f=w3923) -> (s? t:f=w3930:dbl)
            n2219 = Select(t=w3936, s=w3938, f=w3927) -> (s? t:f=w3931:dbl)
            n2220 = call "Volt to I16.vi"("Voltage In"=w3931) -> ("I16 Voltage Out"=w3934:i16)
            n2221 = call "Volt to I16.vi"("Voltage In"=w3930) -> ("I16 Voltage Out"=w3933:i16)
            n2222 = xnode "Read/Write Control"("FPGA VI Reference In"=w3947, "error in"=w3946, "AI to FIFO"=w3943, "APD to FIFO"=w3943, "Start scan (MCL)"=w3943, "AO1"=w3934, "AO2"=w3933) -> ("FPGA VI Reference Out"=w3945:T19, "error out"=w3944:errorcluster)
          }
        }
        "Initial Y" <- w3896
        "Initial X" <- w3895
        n2223 = local write "Tab Control 6"(T3."Imaging" ("Tab Control 6")) -> ()
        "wait to reset values" <- w3897
      }
    }
    n2224 = local read "Trap Pos Elements/DMA read"() -> (w3247:u32)
    n2225 = local read "Trap AI Elements/DMA read"() -> (w3322:u32)
    n2226 = local read "APD Elements/DMA read"() -> (w3288:u32)
    n2227 = xnode "Get APD Data"("FPGA VI Reference In"=w3251, "error in"=w3250, "Number of Elements"=w3288, "Timeout (ms)"=-1) -> ("Data"=w3287:u32[], "Elements Remaining"=→"APD FIFO Elements Remaining":u32)  [unwired: 2 out]
    n2228 = xnode "Invoke Method"("FPGA VI Reference In"=w3251, "error in"=w3250, "Number of Elements"=w3247, "Timeout (ms)"=-1) -> ("Data"=w3210:u16[], "Elements Remaining"=→"Trap Pos FIFO El Remaining":u32)  [unwired: 2 out]
    n2229 = xnode "Get Trap Data"("FPGA VI Reference In"=w3251, "error in"=w3250, "Number of Elements"=w3322, "Timeout (ms)"=-1 ("Timeout")) -> ("FPGA VI Reference Out"=w3144:T19, "error out"=w3143:errorcluster, "Data"=w3211:i16[], "Elements Remaining"=w3453:u32)
    "FIFO El. Rem." <- w3453
    n2230 = local read "Trap AI FIFO Depth"() -> (w3455:u32)
    n2231 = Subtract(x=w3455, y=w3322) -> (x-y=w3454:u32)
    n2232 = Decimate 1D Array(w3210) -> (w3207:u16[], w3209:u16[], w3208:u16[])
    n2233 = Divide(x=w3453, y=w3454) -> (x/y=w3452:dbl)
    "Buffer Status" <- w3452
    n2234 = To Unsigned Long Integer(number=w3207) -> (unsigned 32bit integer=w3206:u32[])
    n2235 = Join Numbers(hi=w3209, lo=w3208) -> ((hi.lo)=w3205:u32[])
    n2236 = Equal?(x=w3452, y=1.0) -> (x = y?=w3450:bool)
    n2237 = Join Numbers(hi=w3206, lo=w3205) -> ((hi.lo)=w3199:u64[])
    n2238 = call "IR AOM word to freq - vec.vi"("Frequency Word In (double vec)"=w3199) -> ("Frequency Out"=w3246:dbl[])
    n2239 = case "Alert buffer overflow" shown="True" w3450 {
      frame False {
      }
      frame True {
        n2240 = call <vilib>:"Beep.vi"() -> ()  [unwired: 3 in, 9 out]
        "Overflow (data lost)" <- TRUE ("Overflow (data lost)")
      }
    }
    n2241 = Decimate 1D Array(w3246) -> (w3245:dbl[], w3244:dbl[])
    n2242 = Build Array(w3245, w3244) -> (w3243:dbl[][])
    n2243 = local read "Trap Sets"() -> (w3321:u32)
    n2244 = case "Deinterlace trap data, average down PSD" shown="2" w3321 {
      tunnel: w3211 -> [w3984 w4049]
      tunnel: [w3981 w4046] -> w3314
      tunnel: [w3984 w4048] -> w3202
      tunnel: "Detector Type" -> [w3983 w4044]
      tunnel: [w3982 w4047] -> w3313
      tunnel: [w3980 w4045] -> w3427
      frame 1, Default {
        n2245 = Divide(x=w3984, y=3276.7) -> (x/y=w3985:dbl[])
        n2246 = Decimate 1D Array(w3985) -> (w3994:dbl[], w3993:dbl[], w3992:dbl[], w3991:dbl[], w3990:dbl[], w3989:dbl[], w3988:dbl[], w3987:dbl[])
        n2247 = case shown="\"IR-QPD + PSD + FB-QPD position\"" w3983 {
          tunnel: w3994 -> [w4018 w4043]
          tunnel: w3993 -> [w4017 w4042]
          tunnel: w3992 -> [w4002 w4020]
          tunnel: w3991 -> [w4003 w4030]
          tunnel: w3990 -> [w4016 w4041]
          tunnel: w3989 -> [w4015 w4040]
          tunnel: w3988 -> [w3999 w4021]
          tunnel: w3987 -> [w3998 w4019]
          tunnel: [w3997 w4027] -> w3982
          tunnel: [w3996 w4026] -> w3981
          tunnel: [w3995 w4025] -> w3980
          frame "IR-QPD + PSD + FB-QPD", Default {
            w3995 = 0  # Channel pattern
            n2248 = Divide(x=w4018, y=w4003) -> (x/y=w4005:dbl[])
            n2249 = Divide(x=w4017, y=w4003) -> (x/y=w4004:dbl[])
            n2250 = Divide(x=w4016, y=w3999) -> (x/y=w4001:dbl[])
            n2251 = Divide(x=w4015, y=w3998) -> (x/y=w4000:dbl[])
            n2252 = Build Array(w4005, w4004, w4003, w4002, w4001, w4000, w3999, w3998) -> (w3996:dbl[][])
            n2253 = Bundle("T1 Y", "T1 X", "T1 Sum", "FB Sum", "PSD Y", "PSD X", "PSD Y Sum", "PSD X Sum") -> (w4014:T40)  [unwired: 1 out]
            n2254 = Cluster To Array(cluster=w4014) -> (array=w3997:string[])
          }
          frame "IR-QPD + PSD + FB-QPD position" {
            w4025 = 3  # Channel pattern
            n2255 = Negate(x=w4021) -> (-x=w4022:dbl[])
            n2256 = Divide(x=w4043, y=w4030) -> (x/y=w4032:dbl[])
            n2257 = Divide(x=w4042, y=w4030) -> (x/y=w4031:dbl[])
            n2258 = Divide(x=w4041, y=w4021) -> (x/y=w4029:dbl[])
            n2259 = Divide(x=w4040, y=w4022) -> (x/y=w4028:dbl[])
            n2260 = Build Array(w4032, w4031, w4030, w4019, w4020, w4029, w4028, w4021) -> (w4026:dbl[][])
            n2261 = Bundle("T1 Y", "T1 X", "T1 Sum", "FB X", "FB Sum", "PSD Y", "PSD X", "PSD Y Sum") -> (w4039:T40)  [unwired: 1 out]
            n2262 = Cluster To Array(cluster=w4039) -> (array=w4027:string[])
          }
        }
      }
      frame 2 {
        n2263 = case shown="\"IR-QPD + PSD + FB-QPD X position\"" w4044 {
          tunnel: w4049 -> [w4111 w4178 w4249]
          tunnel: [w4050 w4169 w4180] -> w4048
          tunnel: [w4077 w4160 w4227] -> w4047
          tunnel: [w4076 w4123 w4194] -> w4046
          tunnel: [w4070 w4158 w4225] -> w4045
          frame "IR-QPD + PSD + FB-QPD", Default {
            w4070 = 1  # Channel pattern
            # "time average x2 the 4th signal and the 4 psd signals (detection laser)"
            # "deinterlace 3 signals from qpd"
            n2264 = Decimate 1D Array(w4111) -> (w4110:i16[], w4109:i16[], w4075:i16[], w4108:i16[], w4098:i16[], w4096:i16[], w4095:i16[], w4093:i16[])
            n2265 = Decimate 1D Array(w4075) -> (w4074:i16[], w4073:i16[])
            n2266 = Decimate 1D Array(w4110) -> (w4107:i16[], w4079:i16[])
            n2267 = Decimate 1D Array(w4109) -> (w4106:i16[], w4104:i16[])
            n2268 = Decimate 1D Array(w4108) -> (w4105:i16[], w4103:i16[])
            n2269 = call "downsample 1D array - double.vi"("Ave N"=2.0, "Array In"=w4098) -> ("Array Out"=w4097:dbl[])  [unwired: 1 out]
            n2270 = call "downsample 1D array - double.vi"("Ave N"=2.0, "Array In"=w4096) -> ("Array Out"=w4078:dbl[])  [unwired: 1 out]
            n2271 = call "downsample 1D array - double.vi"("Ave N"=2.0, "Array In"=w4095) -> ("Array Out"=w4094:dbl[])  [unwired: 1 out]
            n2272 = call "downsample 1D array - double.vi"("Ave N"=2.0, "Array In"=w4093) -> ("Array Out"=w4092:dbl[])  [unwired: 1 out]
            n2273 = Interleave 1D Arrays(w4107, w4106, w4105, w4079, w4104, w4103, w4074, w4073, w4097, w4078, w4094, w4092) -> (w4091:dbl[])
            n2274 = Divide(x=w4091, y=3276.7) -> (x/y=w4090:dbl[])
            n2275 = Decimate 1D Array(w4090) -> (w4089:dbl[], w4088:dbl[], w4087:dbl[], w4086:dbl[], w4085:dbl[], w4084:dbl[], w4072:dbl[], w4071:dbl[], w4083:dbl[], w4082:dbl[], w4081:dbl[], w4080:dbl[])
            n2276 = Divide(x=w4089, y=w4087) -> (x/y=w4057:dbl[])
            n2277 = Divide(x=w4088, y=w4087) -> (x/y=w4056:dbl[])
            n2278 = Divide(x=w4086, y=w4084) -> (x/y=w4055:dbl[])
            n2279 = Divide(x=w4085, y=w4084) -> (x/y=w4054:dbl[])
            n2280 = Divide(x=w4083, y=w4081) -> (x/y=w4053:dbl[])
            n2281 = Divide(x=w4082, y=w4080) -> (x/y=w4052:dbl[])
            n2282 = Build Array(w4057, w4056, w4087, w4055, w4054, w4084, w4072, w4071, w4053, w4052, w4081, w4080) -> (w4076:dbl[][])
            n2283 = Bundle("T1 Y", "T1 X", "T1 Sum", "T2 Y", "T2 X", "T2 Sum", "T1 FB Sum", "T2 FB Sum", "PSD Y", "PSD X", "PSD Y Sum", "PSD X Sum") -> (w4058:T41)  [unwired: 1 out]
            n2284 = To Word Integer(number=w4091) -> (16bit integer=w4050:i16[])
            n2285 = Cluster To Array(cluster=w4058) -> (array=w4077:string[])
          }
          frame "IR-QPD + PSD + FB-QPD X position" {
            w4158 = 2  # Channel pattern
            # "time average x2 the 3 psd signals (detection laser)"
            # "deinterlace 3 signals from qpds"
            n2286 = Decimate 1D Array(w4178) -> (w4177:i16[], w4176:i16[], w4159:i16[], w4175:i16[], w4121:i16[], w4118:i16[], w4115:i16[], w4146:i16[])
            n2287 = Decimate 1D Array(w4159) -> (w4144:i16[], w4142:i16[])
            n2288 = Decimate 1D Array(w4177) -> (w4174:i16[], w4161:i16[])
            n2289 = Decimate 1D Array(w4176) -> (w4173:i16[], w4171:i16[])
            n2290 = Decimate 1D Array(w4175) -> (w4172:i16[], w4170:i16[])
            n2291 = Decimate 1D Array(w4146) -> (w4145:i16[], w4143:i16[])
            n2292 = call "downsample 1D array - I16.vi"("Ave N"=2.0, "Array In"=w4121) -> ("Array Out"=w4119:i16[])  [unwired: 1 in]
            n2293 = call "downsample 1D array - I16.vi"("Ave N"=2.0, "Array In"=w4115) -> ("Array Out"=w4113:i16[])  [unwired: 1 in]
            n2294 = call "downsample 1D array - I16.vi"("Ave N"=2.0, "Array In"=w4118) -> ("Array Out"=w4116:i16[])  [unwired: 1 in]
            n2295 = Interleave 1D Arrays(w4174, w4173, w4172, w4161, w4171, w4170, w4145, w4144, w4143, w4142, w4119, w4116, w4113) -> (w4169:i16[])
            n2296 = Divide(x=w4169, y=3276.7) -> (x/y=w4168:dbl[])
            n2297 = Decimate 1D Array(w4168) -> (w4167:dbl[], w4166:dbl[], w4165:dbl[], w4164:dbl[], w4163:dbl[], w4162:dbl[], w4134:dbl[], w4132:dbl[], w4131:dbl[], w4129:dbl[], w4128:dbl[], w4127:dbl[], w4124:dbl[])
            n2298 = Negate(x=w4124) -> (-x=w4122:dbl[])
            n2299 = Divide(x=w4128, y=w4124) -> (x/y=w4126:dbl[])
            n2300 = Divide(x=w4127, y=w4122) -> (x/y=w4125:dbl[])
            n2301 = Divide(x=w4167, y=w4165) -> (x/y=w4150:dbl[])
            n2302 = Divide(x=w4166, y=w4165) -> (x/y=w4149:dbl[])
            n2303 = Divide(x=w4164, y=w4162) -> (x/y=w4148:dbl[])
            n2304 = Divide(x=w4163, y=w4162) -> (x/y=w4147:dbl[])
            n2305 = Divide(x=w4134, y=w4132) -> (x/y=w4133:dbl[])
            n2306 = Divide(x=w4131, y=w4129) -> (x/y=w4130:dbl[])
            n2307 = Build Array(w4150, w4149, w4165, w4148, w4147, w4162, w4133, w4132, w4130, w4129, w4126, w4125, w4124) -> (w4123:dbl[][])
            n2308 = Bundle("T1 Y", "T1 X", "T1 Sum", "T2 Y", "T2 X", "T2 Sum", "T1 FB X", "T1 FB Sum", "T2 FB X", "T2 FB Sum", "PSD Y", "PSD X", "PSD Y Sum") -> (w4151:T42)  [unwired: 1 out]
            n2309 = Cluster To Array(cluster=w4151) -> (array=w4160:string[])
          }
          frame "IR-QPD + PSD + FB-QPD XY positions" {
            w4225 = 4  # Channel pattern
            # "time average x2 the 3 psd signals (detection laser)"
            # "deinterlace 3 signals from qpds"
            n2310 = Decimate 1D Array(w4249) -> (w4248:i16[], w4247:i16[], w4226:i16[], w4246:i16[], w4192:i16[], w4238:i16[], w4237:i16[], w4214:i16[])
            n2311 = Decimate 1D Array "Feedback Sum"(w4226) -> (w4210:i16[], w4208:i16[])
            n2312 = Decimate 1D Array "QPD Y"(w4248) -> (w4245:i16[], w4228:i16[])
            n2313 = Decimate 1D Array "QPD X"(w4247) -> (w4244:i16[], w4242:i16[])
            n2314 = Decimate 1D Array "Feedback Y"(w4192) -> (w4191:i16[], w4190:i16[])
            n2315 = Decimate 1D Array "QPD Sum"(w4246) -> (w4243:i16[], w4241:i16[])
            n2316 = Decimate 1D Array "Feedback X"(w4214) -> (w4211:i16[], w4209:i16[])
            n2317 = call "downsample 1D array - double.vi"("Ave N"=2.0, "Array In"=w4238) -> ("Array Out"=w4213:dbl[])  [unwired: 1 out]
            n2318 = call "downsample 1D array - double.vi"("Ave N"=2.0, "Array In"=w4237) -> ("Array Out"=w4212:dbl[])  [unwired: 1 out]
            n2319 = Interleave 1D Arrays(w4245, w4244, w4243, w4228, w4242, w4241, w4191, w4211, w4210, w4190, w4209, w4208, w4213, w4212) -> (w4236:dbl[])
            n2320 = Divide(x=w4236, y=3276.7) -> (x/y=w4235:dbl[])
            n2321 = Decimate 1D Array(w4235) -> (w4234:dbl[], w4233:dbl[], w4232:dbl[], w4231:dbl[], w4230:dbl[], w4229:dbl[], w4187:dbl[], w4201:dbl[], w4185:dbl[], w4186:dbl[], w4199:dbl[], w4183:dbl[], w4197:dbl[], w4195:dbl[])
            n2322 = Negate(x=w4195) -> (-x=w4193:dbl[])
            n2323 = Divide(x=w4197, y=w4193) -> (x/y=w4196:dbl[])
            n2324 = Divide(x=w4186, y=w4183) -> (x/y=w4182:dbl[])
            n2325 = Divide(x=w4187, y=w4185) -> (x/y=w4184:dbl[])
            n2326 = Divide(x=w4234, y=w4232) -> (x/y=w4218:dbl[])
            n2327 = Divide(x=w4233, y=w4232) -> (x/y=w4217:dbl[])
            n2328 = Divide(x=w4231, y=w4229) -> (x/y=w4216:dbl[])
            n2329 = Divide(x=w4230, y=w4229) -> (x/y=w4215:dbl[])
            n2330 = Divide(x=w4201, y=w4185) -> (x/y=w4200:dbl[])
            n2331 = Divide(x=w4199, y=w4183) -> (x/y=w4198:dbl[])
            n2332 = Build Array(w4218, w4217, w4232, w4216, w4215, w4229, w4184, w4200, w4185, w4182, w4198, w4183, w4196, w4195) -> (w4194:dbl[][])
            n2333 = Bundle("T1 Y", "T1 X", "T1 Sum", "T2 Y", "T2 X", "T2 Sum", "T1 FB Y", "T1 FB X", "T1 FB Sum", "T2 FB Y", "T2 FB X", "T2 FB Sum", "PSD X", "PSD Y Sum") -> (w4181:T43)  [unwired: 1 out]
            n2334 = To Word Integer(number=w4236) -> (16bit integer=w4180:i16[])
            n2335 = Cluster To Array(cluster=w4181) -> (array=w4227:string[])
          }
        }
      }
    }
    "AI labels" <- w3313
    n2336 = Decimate 1D Array(w3287) -> (w3311:u32[], w3255:u32[])
    n2337 = local read "DMA Update Period (s)"() -> (w3323:dbl)
    n2338 = Build Array(w3311, w3255) -> (w3389:u32[][])
    n2339 = local read "Data Period (s)"() -> (w3161:dbl)
    n2340 = local read "BD 1 Frequency 2 (MHz)"() -> (w3194:dbl)
    n2341 = local read "BD 1 Frequency 1 (MHz)"() -> (w3195:dbl)
    n2342 = Decimate 1D Array(w3202) -> (w3226:i16[], w3225:i16[], w3223:i16[], w3222:i16[])  [unwired: 9 out]
    n2343 = To Double Precision Float(number=w3389) -> (double precision float=w3390:dbl[][])
    n2344 = local read "APD Integration Time (s)"() -> (w3268:dbl)
    n2345 = Multiply(x=w3161, y="Trap Pos. Disp. Downsample") -> (x*y=w3159:dbl)
    n2346 = Divide(x=w3226, y=w3225) -> (x/y=w3227:dbl[])
    n2347 = Divide(x=w3223, y=w3222) -> (x/y=w3224:dbl[])
    n2348 = feedback #6(0.0) -> (w3240:dbl)
    n2349 = Add(x=w3323, y=w3240) -> (x+y=w3429:dbl)
    n2350 = feedback-in #6(w3429) -> ()
    n2351 = local read "AOM X Cal (nm/MHz)"() -> (w3192:dbl)
    n2352 = To Time Stamp(1:w3240) -> (0:w3239:timestamp)
    n2353 = Split 1D Array(array=w3227, index="N El. to Ave.") -> (second subarray=w3230:dbl[])  [unwired: 1 out]
    n2354 = Split 1D Array(array=w3224, index="N El. to Ave.") -> (second subarray=w3229:dbl[])  [unwired: 1 out]
    n2355 = Multiply(x=w3161, y="Trap Disp. Downsample") -> (x*y=w3241:dbl)
    "Display Period (s)" <- w3241
    n2356 = for "Trap AI" {
      tunnel: [w3979] -> w3423 mode=indexing
      tunnel: w3239 -> [w3969]
      tunnel: "Trap Disp. Downsample" -> [w3977]
      tunnel: w3314 -> [w3975] mode=indexing
      tunnel: w3161 -> [w3974]
      tunnel: w3313 -> [w3973] mode=indexing
      tunnel: w3238 -> [w3972]
      tunnel: [w3971] -> w3279 mode=indexing
      tunnel: w3241 -> [w3970]
      workers-P: _ -> [_]
      n2357 = Bundle By Name("Y"=w3975, "dt"=w3974) -> (w3976:waveform(dbl))  [unwired: 1 out]
      n2358 = Set Waveform Attribute(5:w3973, 6:w3972, 7:w3976) -> (3:w3971:waveform(dbl))  [unwired: 1 in, 2 out]
